vi "DAQ_Initialization.vi"(4 "AO Lasers":tag="USB-6363/ao1:3", 6 "AO Pockels":tag="USB-6363/ao0", 7 "DO":tag="USB-6363/port0/line0:3", 8 "error in (no error)":errorcluster, 9 "Counter":tag="USB-6363/ctr0", 10 "Timing source":tag="OnboardClock", 11 "DO | Trigger":tag="/USB-6363/PFI12") -> (0 "error out":errorcluster)   [LabVIEW 2025]
uses:
  <vilib>/DAQmx/create/channels.llb/DAQmx Create Channel (CO-Pulse Generation-Time).vi
  <vilib>/DAQmx/create/channels.llb/DAQmx Create Channel (DO-Digital Output).vi
  <vilib>/DAQmx/configure/trigger.llb/DAQmx Start Trigger (Digital Edge).vi
  <vilib>/DAQmx/configure/timing.llb/DAQmx Timing (Sample Clock).vi
  <resource>/objmgr/daqmx.rc
  <vilib>/DAQmx/create/channels.llb/DAQmx Create Channel (AO-Voltage-Basic).vi
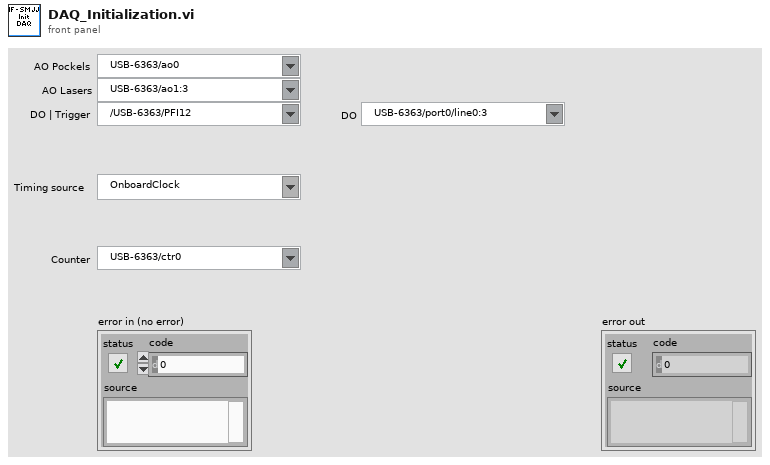
[diagram p1: front panel]
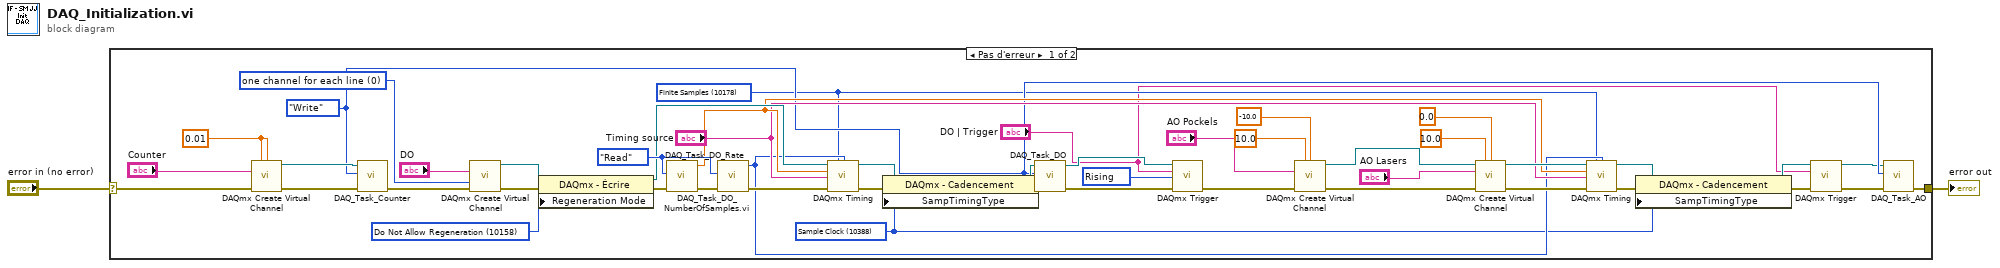
[diagram p0: block diagram]
diagram:
  n1 = case shown="Pas d'erreur" "error in (no error)" {
    selector: "error in (no error)" -> [w28 w51]
    tunnel: [w6 w51] -> w2
    frame No Error {
      w50 = 0 items=["one channel for each line", "one channel for all lines"] ("line grouping")
      w49 = enum16{"Write", "Read"}."Read" ("Action")
      w12 = 10388 items=["Sample Clock"=10388, "Burst Handshake"=12548, "Handshake"=10389, "Implicit"=10451, "On Demand"=10390, "Change Detection"=12504, "Pipelined Sample Clock"=14668] ("SampTimingType")
      w13 = 10178 items=["Finite Samples"=10178, "Continuous Samples"=10123] ("sample mode")
      w39 = 10158 items=["Allow Regeneration"=10097, "Do Not Allow Regeneration"=10158] ("RegenMode")
      w37 = 10280 items=["Rising"=10280, "Falling"=10171] ("edge")
      w36 = 0.01 ("low time")
      w15 = enum16{"Write", "Read"}."Write" ("Action")
      n2 = call-poly <vilib>:"DAQmx Create Virtual Channel.vi"("high time"=w36, "low time"=w36, "counter"="Counter", "error in"=w28) -> ("task out"=w32:refnum<k21>, "error out"=w31:errorcluster)  [unwired: 10 in]
      n3 = call "DAQ_Task_Counter.vi"("error in"=w31, "Action"=w15, "DAQ_Task_Counter"=w32) -> ("error out"=w33:errorcluster)  [unwired: 7 in, 1 out]
      n4 = call-poly <vilib>:"DAQmx Create Virtual Channel.vi"("lines"="DO", "line grouping"=w50, "error in"=w33) -> ("task out"=w41:refnum<k21>, "error out"=w40:errorcluster)  [unwired: 11 in]
      n5 = property class="DAQmx - Écrire"(reference=w41, error in=w40, "Regeneration Mode"=w39) -> (reference out=w38:refnum<k21>, error out=w46:errorcluster)
      n6 = call "DAQ_Task_DO_Rate.vi"("error in"=w46, "Action"=w49) -> ("error out"=w47:errorcluster, "DO_Rate"=w18:dbl)  [unwired: 8 in]
      n7 = call "DAQ_Task_DO_NumberOfSamples.vi.vi"("error in"=w47, "Action"=w49) -> ("error out"=w48:errorcluster, "Samples"=w14:i32)  [unwired: 8 in]
      n8 = call-poly <vilib>:"DAQmx Timing.vi"("task/channels in"=w38, "sample mode"=w13, "samples per channel"=w14, "rate"=w18, "source"="Timing source", "error in"=w48) -> ("task out"=w44:refnum<k21>, "error out"=w43:errorcluster)  [unwired: 8 in]
      n9 = property class="DAQmx - Cadencement"(reference=w44, error in=w43, "SampTimingType"=w12) -> (reference out=w45:refnum<k21>, error out=w42:errorcluster)
      n10 = call "DAQ_Task_DO.vi"("error in"=w42, "Action"=w15, "DAQ_Task_DO"=w45) -> ("error out"=w35:errorcluster, "DAQ_Task_DO"=w34:refnum<k21>)  [unwired: 7 in]
      n11 = call-poly <vilib>:"DAQmx Trigger.vi"("task/channels in"=w34, "source"="DO | Trigger", "edge"=w37, "error in"=w35) -> ("error out"=w27:errorcluster)  [unwired: 10 in, 1 out]
      n12 = call-poly <vilib>:"DAQmx Create Virtual Channel.vi"("maximum value"=10.0, "minimum value"=-10.0, "physical channels"="AO Pockels", "error in"=w27) -> ("task out"=w23:refnum<k21>, "error out"=w3:errorcluster)  [unwired: 10 in]
      n13 = call-poly <vilib>:"DAQmx Create Virtual Channel.vi"("task in"=w23, "maximum value"=10.0, "minimum value"=0.0, "physical channels"="AO Lasers", "error in"=w3) -> ("task out"=w19:refnum<k21>, "error out"=w16:errorcluster)  [unwired: 9 in]
      n14 = call-poly <vilib>:"DAQmx Timing.vi"("task/channels in"=w19, "sample mode"=w13, "samples per channel"=w14, "rate"=w18, "source"="Timing source", "error in"=w16) -> ("task out"=w4:refnum<k21>, "error out"=w5:errorcluster)  [unwired: 8 in]
      n15 = property class="DAQmx - Cadencement"(reference=w4, error in=w5, "SampTimingType"=w12) -> (reference out=w11:refnum<k21>, error out=w10:errorcluster)
      n16 = call-poly <vilib>:"DAQmx Trigger.vi"("task/channels in"=w11, "source"="DO | Trigger", "error in"=w10) -> ("task out"=w8:refnum<k21>, "error out"=w7:errorcluster)  [unwired: 11 in]
      n17 = call "DAQ_Task_AO.vi"("error in"=w7, "Action"=w15, "DAQ_Task_DO"=w8) -> ("error out"=w6:errorcluster)  [unwired: 7 in, 1 out]
    }
    frame Error {
    }
  }
  "error out" <- w2
